vi "Bytes_To_Bits.vi"(0 "Data":string, 5 "offset (0)":i32=4, 7 "length (rest)":i32=2) -> (8 "output cluster":T1)   [LabVIEW 2021]
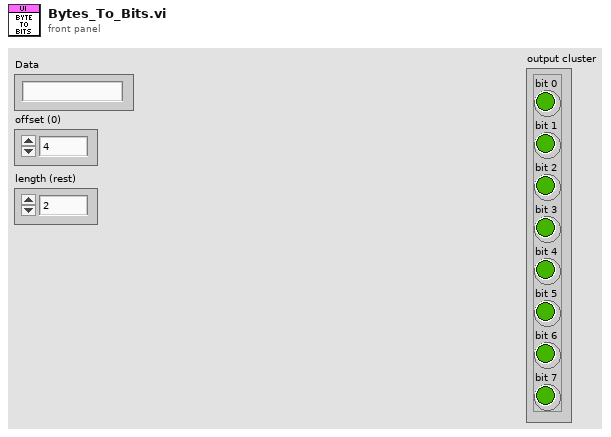
[diagram p1: front panel]
types:
  T1 = cluster{"bit 0":bool, "bit 1":bool, "bit 2":bool, "bit 3":bool, "bit 4":bool, "bit 5":bool, "bit 6":bool, "bit 7":bool}
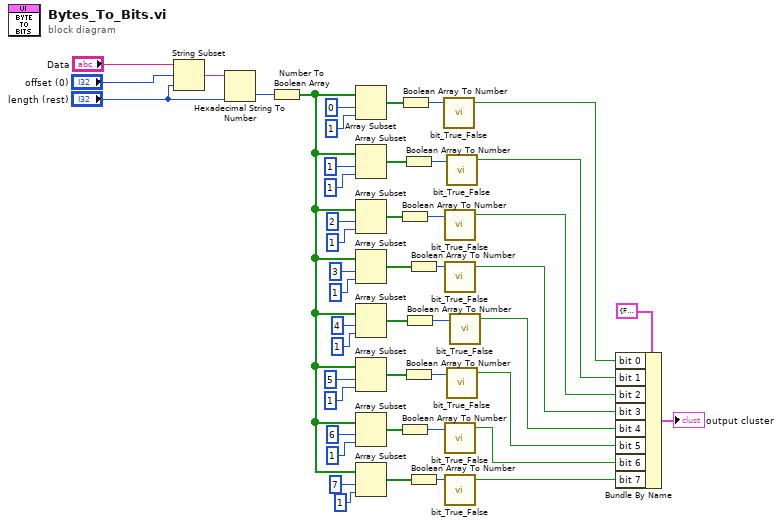
[diagram p0: block diagram]
diagram:
  n1 = String Subset(string="Data", offset (0)="offset (0)", length (rest)="length (rest)") -> (substring=w47:string)
  n2 = Hexadecimal String To Number(string=w47, default (0uL)="length (rest)") -> (number=w48:i32)  [unwired: 1 in, 1 out]
  n3 = Number To Boolean Array(number=w48) -> (Boolean array=w13:bool[])
  n4 = Array Subset(array=w13, index=0, length=1) -> (w26:bool[])
  n5 = Array Subset(array=w13, index=1, length=1) -> (w30:bool[])
  n6 = Array Subset(array=w13, index=2, length=1) -> (w33:bool[])
  n7 = Array Subset(array=w13, index=3, length=1) -> (w37:bool[])
  n8 = Array Subset(array=w13, index=4, length=1) -> (w34:bool[])
  n9 = Array Subset(array=w13, index=5, length=1) -> (w22:bool[])
  n10 = Array Subset(array=w13, index=6, length=1) -> (w19:bool[])
  n11 = Array Subset(array=w13, index=7, length=1) -> (w18:bool[])
  n12 = Boolean Array To Number(Boolean array=w33) -> (number=w42:u32)
  n13 = Boolean Array To Number(Boolean array=w19) -> (number=w15:u32)
  n14 = Boolean Array To Number(Boolean array=w26) -> (number=w40:u32)
  n15 = Boolean Array To Number(Boolean array=w30) -> (number=w41:u32)
  n16 = Boolean Array To Number(Boolean array=w22) -> (number=w16:u32)
  n17 = Boolean Array To Number(Boolean array=w34) -> (number=w44:u32)
  n18 = Boolean Array To Number(Boolean array=w37) -> (number=w43:u32)
  n19 = Boolean Array To Number(Boolean array=w18) -> (number=w14:u32)
  n20 = call "bit_True_False.vi"("number"=w40) -> ("True?"=w2:bool)  [unwired: 4 in]
  n21 = call "bit_True_False.vi"("number"=w42) -> ("True?"=w4:bool)  [unwired: 4 in]
  n22 = call "bit_True_False.vi"("number"=w43) -> ("True?"=w5:bool)  [unwired: 4 in]
  n23 = call "bit_True_False.vi"("number"=w15) -> ("True?"=w8:bool)  [unwired: 4 in]
  n24 = call "bit_True_False.vi"("number"=w14) -> ("True?"=w9:bool)  [unwired: 4 in]
  n25 = call "bit_True_False.vi"("number"=w41) -> ("True?"=w3:bool)  [unwired: 4 in]
  n26 = call "bit_True_False.vi"("number"=w16) -> ("True?"=w7:bool)  [unwired: 4 in]
  n27 = call "bit_True_False.vi"("number"=w44) -> ("True?"=w6:bool)  [unwired: 4 in]
  n28 = Bundle By Name(cluster=T1 {"bit 0"=FALSE, "bit 1"=FALSE, "bit 2"=FALSE, "bit 3"=FALSE, "bit 4"=FALSE, "bit 5"=FALSE, "bit 6"=FALSE, "bit 7"=FALSE}, "bit 0"=w2, "bit 1"=w3, "bit 2"=w4, "bit 3"=w5, "bit 4"=w6, "bit 5"=w7, "bit 6"=w8, "bit 7"=w9) -> (→"output cluster":T1)
